vi "ex_Vertical Cursors.vi"(6 "X Scale Name":string, 8 "x2":dbl=nan format="%0.2f", 9 "x":dbl=nan format="%0.2f", 11 "WFGraph Refnum":refnum<vi>) -> (0 "error out":errorcluster)   [LabVIEW 2020]
doc: "Sets up two vertical cursors on a waveform graph."
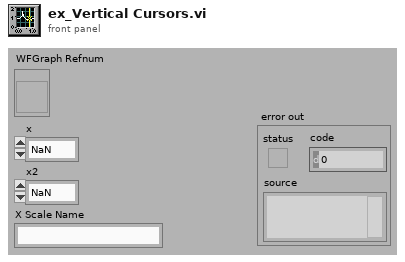
[diagram p1: front panel]
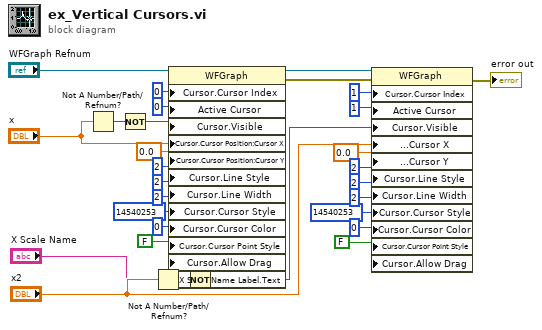
[diagram p0: block diagram]
diagram:
  n1 = Not A Number/Path/Refnum?(number/path/refnum="x") -> (NaN/Path/Refnum?=w4:bool)
  n2 = Not(x=w4) -> (.not. x?=w2:bool)
  n3 = Not A Number/Path/Refnum?(number/path/refnum="x2") -> (NaN/Path/Refnum?=w7:bool)
  n4 = property class="WFGraph"(reference="WFGraph Refnum", "Cursor.Cursor Index"=0, "Active Cursor"=u32 0, "Cursor.Visible"=w2, "Cursor.Cursor Position:Cursor X"="x", "Cursor.Cursor Position:Cursor Y"=0.0, "Cursor.Line Style"=u8 2, "Cursor.Line Width"=u8 2, "Cursor.Cursor Style"=u8 2, "Cursor.Cursor Color"=u32 14540253, "Cursor.Cursor Point Style"=u8 0, "Cursor.Allow Drag"=FALSE, "X Scale.Name Label.Text"="X Scale Name") -> (reference out=w12:refnum<vi>, error out=w11:errorcluster)  [unwired: 1 in]
  n5 = Not(x=w7) -> (.not. x?=w5:bool)
  n6 = property class="WFGraph"(reference=w12, error in=w11, "Cursor.Cursor Index"=1, "Active Cursor"=u32 1, "Cursor.Visible"=w5, "Cursor.Cursor Position:Cursor X"="x2", "Cursor.Cursor Position:Cursor Y"=0.0 ("Cursor.Cursor Position:Cursor X"), "Cursor.Line Style"=u8 2, "Cursor.Line Width"=u8 2, "Cursor.Cursor Style"=u8 2, "Cursor.Cursor Color"=u32 14540253, "Cursor.Cursor Point Style"=u8 0, "Cursor.Allow Drag"=FALSE) -> (error out=→"error out":errorcluster)  [unwired: 1 out]
